vi "CreateHTML.vi"(0 "reference in":refnum<class "Object.lvclass">, 2 "VI Name":string, 5 "error in (no error)":errorcluster) -> (13 "script dependencies":string[](array[string]), 14 "reference out":refnum<class "Object.lvclass">, 15 "HTML":string, 16 "js variables":string, 17 "js code for controls":string, 18 "js code for indicators":string, 19 "error out":errorcluster)   [LabVIEW 2014, in "Object.lvclass"]
uses:
  Object.lvclass
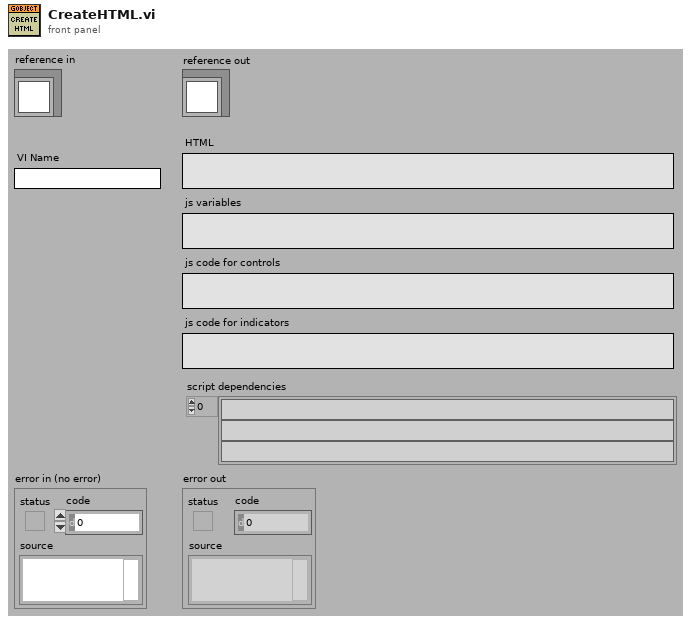
[diagram p1: front panel]
types:
  T1 = typedef "Object.lvclass/Attributes.ctl" = cluster{"UID":i32, "Type":string, "Coordinates":T2, "Reference":refnum<vi>}
  T2 = typedef "Object.lvclass/Coordinates.ctl" = cluster{"Left":i32, "Top":i32, "Height":u32, "Width":u32}
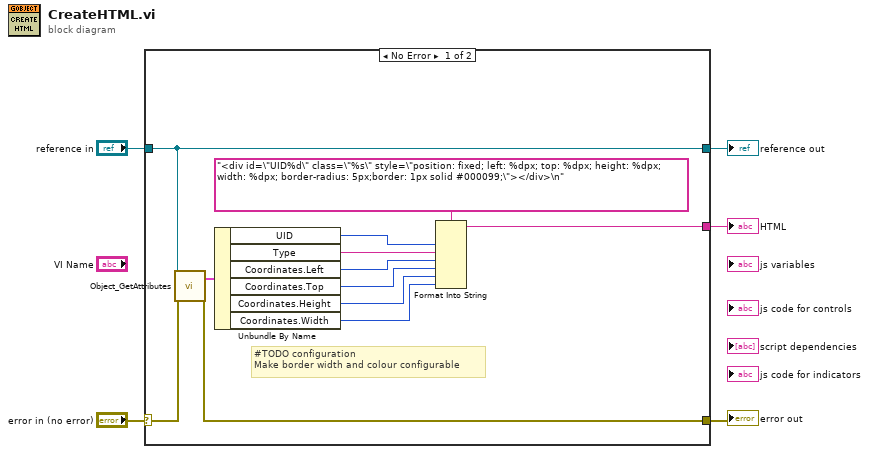
[diagram p0: block diagram]
diagram:
  n1 = case shown="No Error" "error in (no error)" {
    selector: "error in (no error)" -> [w17 w19]
    tunnel: [w16 w19] -> w4
    tunnel: [w6 w18] -> w2
    tunnel: "reference in" -> [w6 w18]
    tunnel: [w7 _] -> w1
    frame No Error {
      # "#TODO configuration\nMake border width and colour configurable"
      n2 = call "Object_GetAttributes.vi"("reference in"=w6, "error in (no error)"=w17) -> ("Data"=w14:T1, "error out"=w16:errorcluster)  [unwired: 14 in, 2 out]
      n3 = Unbundle By Name(w14) -> ("UID"=w13:i32, "Type"=w12:string, "Coordinates.Left"=w11:i32, "Coordinates.Top"=w10:i32, "Coordinates.Height"=w9:u32, "Coordinates.Width"=w8:u32)
      n4 = Format Into String(format string="<div id=\"UID%d\" class=\"%s\" style=\"position: fixed; left: %dpx; top: %dpx; height: %dpx; width: %dpx; border-radius: 5px;border: 1px solid #000099;\"></div>\n", w13, w12, w11, w10, w9, w8) -> (resulting string=w7:string)  [unwired: 2 in, 1 out]
    }
    frame Error {
    }
  }
  "error out" <- w4
  "reference out" <- w2
  "HTML" <- w1
